vi "INI read HW section.vi"(8 "error in (no error)":T1) -> (0 "error out":T1, 1 "timing_class":string, 2 "instr_mode":T2=enum."BB", 3 "instr_class":string, 4 "auto_init":bool)   [LabVIEW 2019, in "Shared.lvlib"]
uses:
  Shared.lvlib
  mmWave instrument_class/Instrument mode.ctl
  System GV.vi
  <vilib>/Utility/error.llb/Error Cluster From Error Code.vi
  <vilib>/ErrorRing/Error Ring.xnode
  <vilib>/Utility/config.llb/NI_LVConfig.lvlib
  mmWave instrument_class/mmWave instrument.lvclass
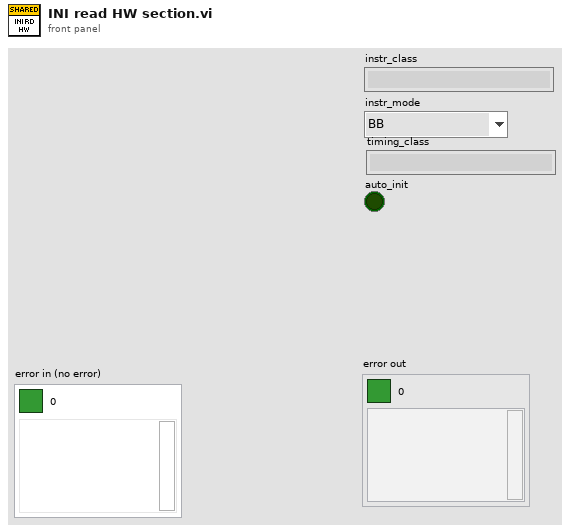
[diagram p1: front panel]
types:
  T1 = cluster{"Boolean Round":bool, "code":i32, "source":string}
  T2 = typedef "mmWave instrument.lvclass/Instrument mode.ctl" = enum16{"RF", "IF", "BB"}
  T3 = cluster{"instr_class":string, "instr_mode":T2, "timing_class":string, "auto_init":bool}
  T4 = typedef "NI_LVConfig.lvlib/Config Data RefNum.ctl" = refnum<k1>
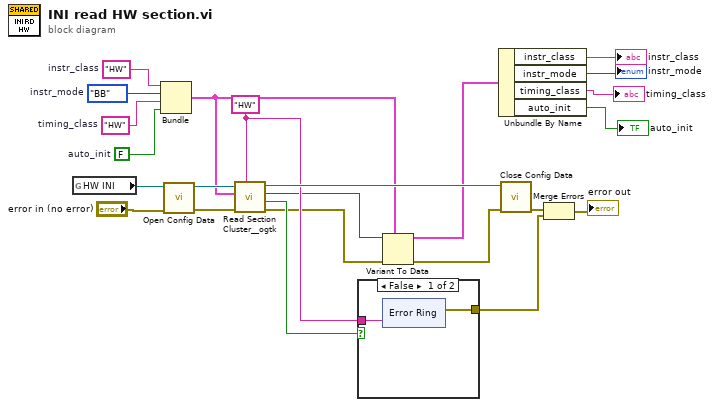
[diagram p0: block diagram]
diagram:
  w2 = FALSE  # auto_init
  w4 = "HW"  # timing_class
  w18 = "HW"  # instr_class
  w19 = Instrument_mode."BB"  # instr_mode
  w16 = "HW" ("section (optional)")
  n1 = global read "System GV.vi" "HW INI"() -> (w20:path)
  n2 = Bundle("instr_class"=w18, "instr_mode"=w19, "timing_class"=w4, "auto_init"=w2) -> (w12:T3)  [unwired: 1 in]
  n3 = call <vilib>:"Open Config Data.vi"("error in (no error)"="error in (no error)", "configuration file path"=w20) -> ("error out"=w21:errorcluster, "refnum"=w23:T4)  [unwired: 7 in, 1 out]
  n4 = call <userlib>:"Read Section Cluster__ogtk.vi"("section (optional)"=w16, "error in (no error)"=w21, "Section Formatted Cluster Type"=w12, "refnum"=w23) -> ("error out"=w14:errorcluster, "all found?"=w17:bool, "Section Formatted Cluster"=w15:variant, "dup refnum"=w22:T4)  [unwired: 3 in, 1 out]
  n5 = case shown="False" w17 {
    tunnel: w16 -> [w25 _]
    tunnel: [w24 _] -> w7
    frame False {
      n6 = xnode "Error Ring"("parameter 0"=w25) -> ("error out"=w24:errorcluster)
    }
    frame True {
    }
  }
  n7 = Variant To Data(error in=w14, type=w12, Variant=w15) -> (data=w11:T3, error out=w13:errorcluster)
  n8 = Unbundle By Name(w11) -> ("instr_class"=→"instr_class":string, "instr_mode"=→"instr_mode":T2, "timing_class"=→"timing_class":string, "auto_init"=→"auto_init":bool)
  n9 = call <vilib>:"Close Config Data.vi"("error in (no error)"=w13, "refnum"=w22) -> ("error out"=w8:errorcluster)  [unwired: 8 in, 1 out]
  n10 = Merge Errors(w8, w7) -> (→"error out":errorcluster)
